vi "serialize.vi"(8 "error in":errorcluster, 11 "Results":T1[](array[typedef])) -> (0 "error out":errorcluster, 3 "serialized results":string)   [LabVIEW 2014, in "VIA-Checkstyle.lvlib"]
uses:
  VIA-Checkstyle.lvlib
  xml format - file.ctl
  xml format - error.ctl
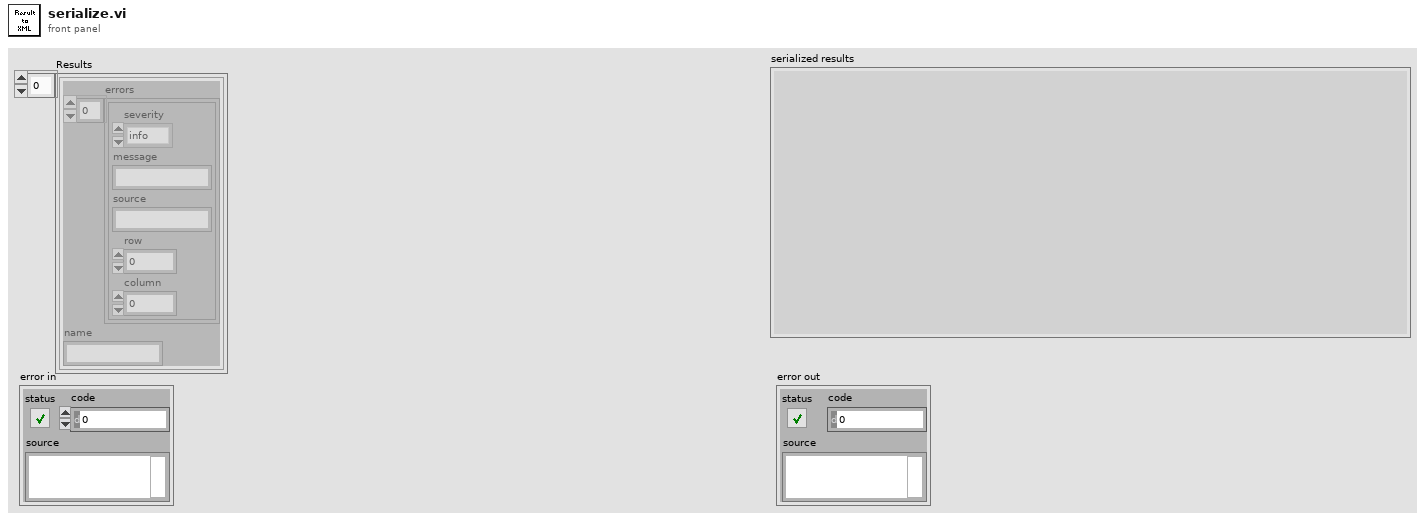
[diagram p1: front panel]
types:
  T1 = typedef "VIA-Checkstyle.lvlib/xml format - file.ctl" = cluster{"errors":T2[], "name":string}
  T2 = typedef "VIA-Checkstyle.lvlib/xml format - error.ctl" = cluster{"severity":enum16{"info", "warning", "error"}, "message":string, "source":string, "row":i32, "column":i32}
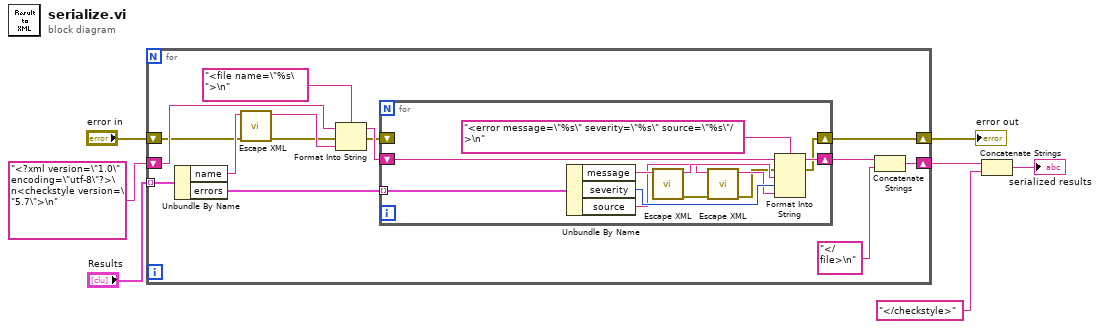
[diagram p0: block diagram]
diagram:
  n1 = for {
    tunnel: "Results" -> [w21] mode=indexing
    shift-right: [w16] -> w1
    shift-left: "error in" -> [w9]
    shift-right: [w12] -> w5
    shift-left: "<?xml version=\"1.0\" encoding=\"utf-8\"?>\n<checkstyle version=\"5.7\">\n" -> [w15]
    n2 = Unbundle By Name(w21) -> ("name"=w11:string, "errors"=w19:T2[])
    n3 = call <vilib>:"Escape XML.vi"("error in (no error)"=w9, "XML String In"=w11) -> ("error out"=w8:errorcluster, "XML String Out"=w10:string)  [unwired: 8 in]
    n4 = Format Into String(format string="<file name=\"%s\">\n", initial string=w15, error in=w8, w10) -> (resulting string=w18:string, error out=w17:errorcluster)
    n5 = for {
      tunnel: w19 -> [w33] mode=indexing
      shift-right: [w31] -> w14
      shift-left: w18 -> [w32]
      shift-right: [w30] -> w16
      shift-left: w17 -> [_]
      n6 = Unbundle By Name(w33) -> ("message"=w26:string, "severity"=w28:enum16{"info", "warning", "error"}, "source"=w24:string)
      n7 = call <vilib>:"Escape XML.vi"("XML String In"=w26) -> ("error out"=w27:errorcluster, "XML String Out"=w25:string)  [unwired: 9 in]
      n8 = call <vilib>:"Escape XML.vi"("error in (no error)"=w27, "XML String In"=w24) -> ("error out"=w22:errorcluster, "XML String Out"=w23:string)  [unwired: 8 in]
      n9 = Format Into String(format string="<error message=\"%s\" severity=\"%s\" source=\"%s\"/>\n", initial string=w32, error in=w22, w25, w28, w23) -> (resulting string=w31:string, error out=w30:errorcluster)
    }
    n10 = Concatenate Strings(w14, "</file>\n" ("string")) -> (w12:string)
  }
  "error out" <- w1
  n11 = Concatenate Strings(w5, "</checkstyle>") -> (→"serialized results":string)
